vi "LWXPS_GPIODigitalSet.vi"(0 "XPS Reference IN":refnum<k24>, 5 "GPIO Name":string, 7 "Mask":u16, 9 "Digital Output Value":u16, 11 "LabVIEW error IN":errorcluster) -> (4 "XPS Reference OUT":refnum<k24>, 6 "Returned error code":i32, 8 "XPS Error String":string, 15 "LabVIEW error OUT":errorcluster)   [LabVIEW 2014]
uses:
  D:/XPSQ8_LabView_Library/Development/Source/Dll/Newport.XPS.CommandInterface.dll
  Dll/Newport.XPS.CommandInterface.dll
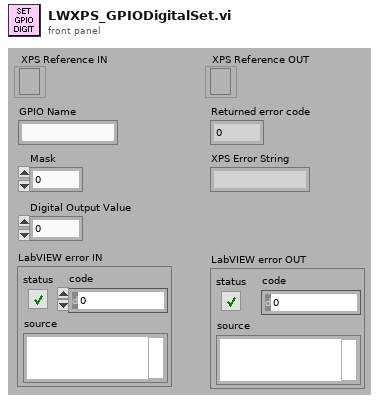
[diagram p1: front panel]
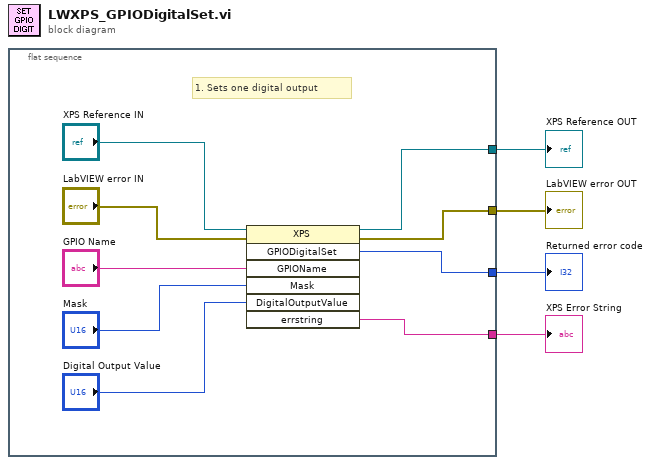
[diagram p0: block diagram]
diagram:
  n1 = flat-sequence {
    tunnel: [w10] -> w4
    tunnel: [w13] -> w3
    tunnel: [w11] -> w2
    tunnel: [w7] -> w1
    frame #0 {
      # "1. Sets one digital output"
      n2 = invoke class="XPS" method="GPIODigitalSet"(reference="XPS Reference IN", error in="LabVIEW error IN", "GPIOName"="GPIO Name", "Mask"="Mask", "DigitalOutputValue"="Digital Output Value") -> (reference out=w10:refnum<k24>, error out=w13:errorcluster, "GPIODigitalSet"=w11:i32, "errstring"=w7:string)  [unwired: 2 in, 3 out]
    }
  }
  "XPS Reference OUT" <- w4
  "LabVIEW error OUT" <- w3
  "Returned error code" <- w2
  "XPS Error String" <- w1
